vi "New ExcuseNote.vi"(6 "CurWeek(0)":i32, 8 "error in (no error)":errorcluster, 9 "Name(\"\")":string, 10 "ID(\"\")":string, 11 "ExcuseNote in":refnum<class "ExcuseNote.lvclass">) -> (0 "error out":errorcluster, 3 "ExcuseNote out":refnum<class "ExcuseNote.lvclass">)   [LabVIEW 2015, in "ExcuseNote.lvclass"]
uses:
  ExcuseNote.lvclass
  ExcuseNote.lvclass/ExcuseNote.ctl
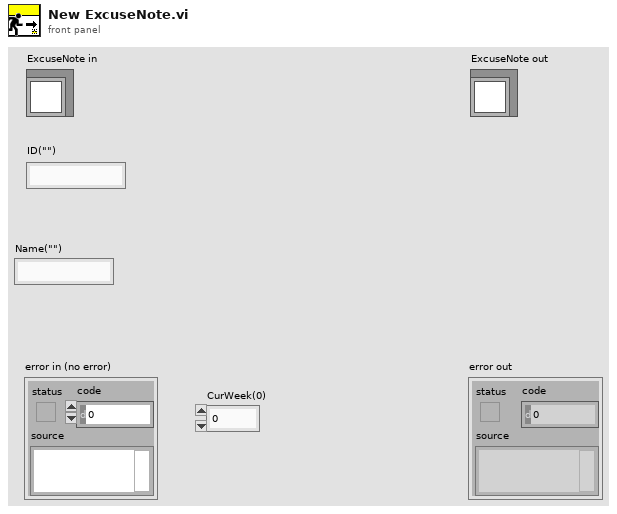
[diagram p1: front panel]
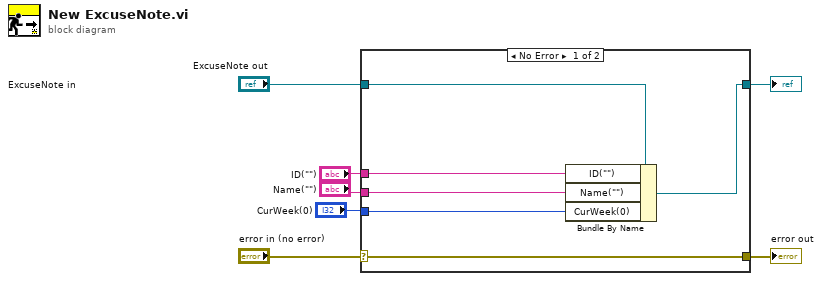
[diagram p0: block diagram]
diagram:
  n1 = case shown="No Error" "error in (no error)" {
    selector: "error in (no error)" -> [w13 w14]
    tunnel: [w13 w14] -> w6
    tunnel: [w11 w15] -> w4
    tunnel: "ExcuseNote in" -> [w12 w15]
    tunnel: "ID(\"\")" -> [w10 _]
    tunnel: "Name(\"\")" -> [w9 _]
    tunnel: "CurWeek(0)" -> [w8 _]
    frame No Error {
      n2 = Bundle By Name(cluster=w12, "ID(\"\")"=w10, "Name(\"\")"=w9, "CurWeek(0)"=w8) -> (w11:refnum<class "ExcuseNote.lvclass">)
    }
    frame Error {
    }
  }
  "error out" <- w6
  "ExcuseNote out" <- w4
